vi "CRYConvert Font.vi"(10 "Font In":T3) -> (1 "[user-specified font]":T1={"Font Name:"="", "Size"=12, "Strikeout?"=FALSE, "Italic?"=FALSE, "Underline?"=FALSE, "Outline?"=FALSE, "Shadow?"=FALSE, "Bold?"=FALSE}, 2 "Control Font":T2)   [LabVIEW 2013]
uses:
  Typedef Control/CRYText Format.ctl
  <vilib>/Utility/miscctls.llb/LVFontTypeDef.ctl
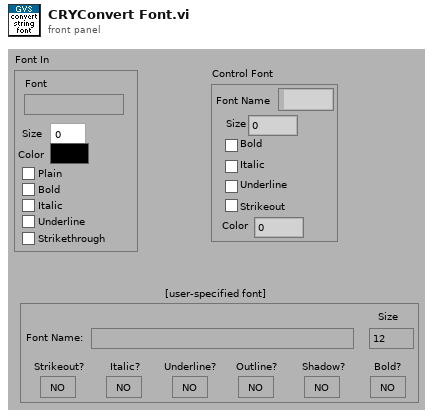
[diagram p1: front panel]
types:
  T1 = cluster{"Font Name:":string, "Size":i16, "Strikeout?":bool, "Italic?":bool, "Underline?":bool, "Outline?":bool, "Shadow?":bool, "Bold?":bool}
  T2 = typedef "LVFontTypeDef.ctl" = cluster{"Font Name":string, "Size":u16, "Bold":bool, "Italic":bool, "Underline":bool, "Strikeout":bool, "Color":u32}
  T3 = typedef "CRYText Format.ctl" = cluster{"Size":u32, "Plain":bool, "Bold":bool, "Italic":bool, "Underline":bool, "Strikethrough":bool, "Color":u32, "Font":string}
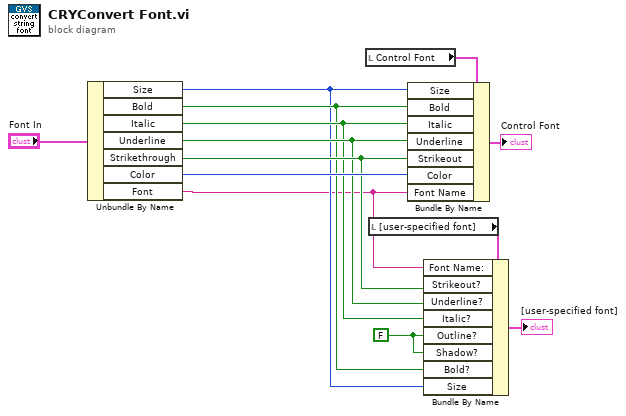
[diagram p0: block diagram]
diagram:
  w4 = FALSE ("Shadow?")
  n1 = Unbundle By Name("Font In") -> ("Size"=w3:u32, "Bold"=w5:bool, "Italic"=w6:bool, "Underline"=w7:bool, "Strikethrough"=w8:bool, "Color"=w11:u32, "Font"=w1:string)
  n2 = local read "Control Font"() -> (w10:T2)
  n3 = local read "[user-specified font]"() -> (w9:T1)
  n4 = Bundle By Name(cluster=w10, "Size"=w3, "Bold"=w5, "Italic"=w6, "Underline"=w7, "Strikeout"=w8, "Color"=w11, "Font Name"=w1) -> (→"Control Font":T2)
  n5 = Bundle By Name(cluster=w9, "Font Name:"=w1, "Strikeout?"=w8, "Underline?"=w7, "Italic?"=w6, "Outline?"=w4, "Shadow?"=w4, "Bold?"=w5, "Size"=w3) -> (→"[user-specified font]":T1)
